vi "ARITHMET.vi"() -> ()   [LabVIEW 2011]
panel:
  out "DIVISION":dbl
  in  "INPUT2":dbl
  in  "INPUT1 4":dbl
  out "MULTI":dbl
  in  "INPUT2":dbl
  in  "INPUT1 3":dbl
  out "SUBTRACT":dbl
  in  "INPUT2":dbl
  in  "INPUT1 2":dbl
  out "ADD":dbl
  in  "INPUT2":dbl
  in  "INPUT1":dbl
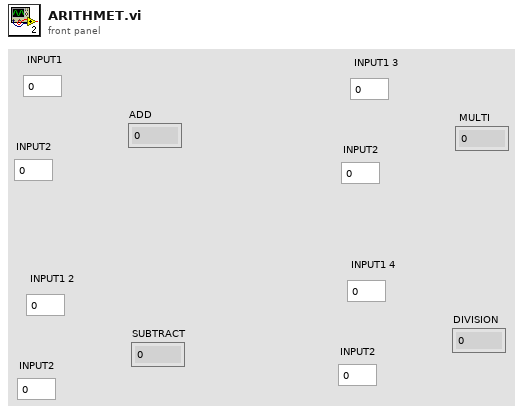
[diagram p1: front panel]
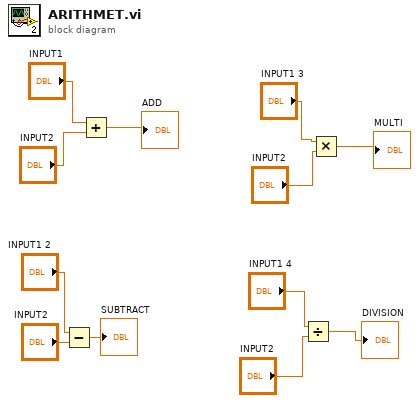
[diagram p0: block diagram]
diagram:
  n1 = Subtract(x="INPUT1 2", y="INPUT2") -> (x-y=→"SUBTRACT":dbl)
  n2 = Add(x="INPUT1", y="INPUT2") -> (x+y=→"ADD":dbl)
  n3 = Divide(x="INPUT1 4", y="INPUT2") -> (x/y=→"DIVISION":dbl)
  n4 = Multiply(x="INPUT1 3", y="INPUT2") -> (x*y=→"MULTI":dbl)
